vi "Begin.vi"() -> (0 "error out":errorcluster)   [LabVIEW 2013]
doc: "Called before other user functions, this VI is expected to open initial I/O refnums, load in file data, and do all program initialization. Notice that the <B>error out</B> terminal is simply used for data flow. Wiring it to other structures or subVIs ensures that this VI runs first."
uses:
  <vilib>/Rock Robotics/WPI/DriverStation/WPI_DriverStationRobotMode2.ctl
  DBNameEnum.ctl
  <vilib>/Rock Robotics/WPI/SafetyOutput/WPI_SafetyOutputConfigMenu.ctl
  <vilib>/Rock Robotics/WPI/Joystick/WPI_JoystickDeviceEnum.ctl
  RefnameEnum.ctl
  SingleSolenoidAction.ctl
  RollerAction.ctl
  TankDriveAction.ctl
  DoubleSolenoidAction.ctl
  CollectorAction.ctl
  <vilib>/Rock Robotics/WPI/Solenoid/WPI_SolenoidChannel.ctl
  <vilib>/Rock Robotics/SystemInterfaces/Typedef/FPGA_TypedefSolenoidModule.ctl
  <vilib>/Rock Robotics/SystemInterfaces/DIO/FPGA_DIOPWMChannel.ctl
  <vilib>/Rock Robotics/SystemInterfaces/Typedef/FPGA_TypedefDigitalModule.ctl
  <vilib>/Rock Robotics/SystemInterfaces/DIO/FPGA_DIOChannel.ctl
  <vilib>/Rock Robotics/SystemInterfaces/DIO/FPGA_DIORelayChannel.ctl
  <vilib>/Rock Robotics/WPI/Relay/WPI_RelayDirection.ctl
  <vilib>/Rock Robotics/SystemInterfaces/AI/FPGA_AIChannel.ctl
  SonarAction.ctl
  <vilib>/Rock Robotics/SystemInterfaces/Typedef/FPGA_TypedefAnalogModule.ctl
  Example_Code/PressureSensor/PressureSensorAction.ctl
  Robot Global Data.vi
  <vilib>/Rock Robotics/WPI/Solenoid/WPI_SolenoidOpenSingle.vi
  <vilib>/Rock Robotics/WPI/MotorControl/WPI_MotorControlOpen Talon.vi
  <vilib>/Rock Robotics/WPI/RobotDrive/WPI_RobotDriveOpen4MotorWithTalon.vi
  <vilib>/Rock Robotics/WPI/Compressor/WPI_CompressorGetSetRefNum.vi
panel:
  in  "Version":string="TF 2.3.2"
  # "SET AS DEFAULT"
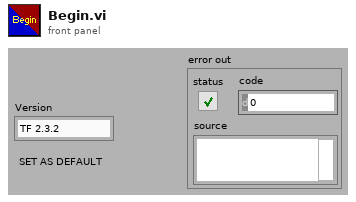
[diagram p1: front panel]
types:
  T1 = typedef "PressureSensorAction.ctl" = enum16{"Init", "ReadValue", "Disable"}
  T2 = typedef "FPGA_AIChannel.ctl" = enum8{"AI 1", "AI 2", "AI 3", "AI 4", "AI 5", "AI 6", "AI 7", "AI 8", "Invalid"}
  T3 = typedef "FPGA_TypedefAnalogModule.ctl" = enum16{"Analog Module 1", "Analog Module 2"}
  T4 = typedef "FPGA_DIOChannel.ctl" = enum8{"DIO 1", "DIO 2", "DIO 3", "DIO 4", "DIO 5", "DIO 6", "DIO 7", "DIO 8", "DIO 9", "DIO 10", "DIO 11", "DIO 12", "DIO 13", "DIO 14", "Invalid"}
  T5 = typedef "FPGA_DIOPWMChannel.ctl" = enum8{"PWM 1", "PWM 2", "PWM 3", "PWM 4", "PWM 5", "PWM 6", "PWM 7", "PWM 8", "PWM 9", "PWM 10", "Invalid"}
  T6 = typedef "SonarAction.ctl" = enum16{"Init", "ReadValue", "Disable"}
  T7 = typedef "WPI_RelayDirection.ctl" = enum16{"Both directions", "Forward only", "Reverse only"}
  T8 = typedef "FPGA_DIORelayChannel.ctl" = enum8{"Relay 1", "Relay 2", "Relay 3", "Relay 4", "Relay 5", "Relay 6", "Relay 7", "Relay 8", "Invalid"}
  T9 = typedef "WPI_SolenoidChannel.ctl" = enum8{"Solenoid 1", "Solenoid 2", "Solenoid 3", "Solenoid 4", "Solenoid 5", "Solenoid 6", "Solenoid 7", "Solenoid 8", "Invalid"}
  T10 = typedef "FPGA_TypedefSolenoidModule.ctl" = enum16{"Solenoid Module 1", "Solenoid Module 2"}
  T11 = typedef "FPGA_TypedefDigitalModule.ctl" = enum16{"Digital Module 1", "Digital Module 2"}
  T12 = typedef "SingleSolenoidAction.ctl" = enum16{"Init", "SetState", "Disable"}
  T13 = typedef "CollectorAction.ctl" = enum16{"Init", "Raise", "Lower", "Stop", "GetStatus"}
  T14 = typedef "DoubleSolenoidAction.ctl" = enum16{"Init", "Middle", "In", "Out"}
  T15 = typedef "TankDriveAction.ctl" = enum16{"Init", "LinearDrive", "SetValue", "Disable"}
  T16 = typedef "RefnameEnum.ctl" = enum16{"TankDrive", "Controller1", "Controller2", "SonicShifter", "Compressor"}
  T17 = typedef "RollerAction.ctl" = enum16{"Init", "Off", "Forward", "Reverse"}
  T18 = typedef "WPI_JoystickDeviceEnum.ctl" = enum16{"USB 1", "USB 2", "USB 3", "USB 4", "Kinect 1", "Kinect 2"}
  T19 = typedef "WPI_SafetyOutputConfigMenu.ctl" = enum16{"Enable", "Disable"}
  T20 = typedef "DBNameEnum.ctl" = enum16{"Version"}
  T21 = typedef "WPI_DriverStationRobotMode2.ctl" = enum16{"Autonomous Disabled", "Autonomous Enabled", "Teleop Disabled", "Teleop Enabled", "Timeout", "Finish", "Test Disabled", "Test Enabled"}
  T22 = typedef "WPI_JoystickDevRef.ctl" = cluster{"Device":T18}
  T23 = typedef "WPI_RobotDriveDevRef.ctl" = cluster{"DevStatus":errorcluster, "Motors[]":T24[], "Square Inputs":bool, "Max Output":dbl, "Isochronous":bool}
  T24 = typedef "WPI_MotorControlDeviceRef.ctl" = cluster{"DeviceStatus":errorcluster, "Type":enum16{"PWM", "CAN"}, "PWM":cluster{"Digital Module":T11, "PWM Channel":T5, "DeadBand":T25}, "CAN":cluster{"Device Number":u8, "Control Mode":T26, "Semaphore":T27, "Max Vout":dbl}, "Invert":bool, "TransformRef":T28, "InvTransformRef":T28}
  T25 = typedef "WPI_PWMDeadband.ctl" = cluster{"Name":string, "maxPositivePwm":i32, "minPositivePwm":i32, "centerPwm":i32, "maxNegativePwm":i32, "minNegativePwm":i32, "angularRange":u16}
  T26 = typedef "WPI_CANJaguar_ControlMode.ctl" = enum8{"Percent VBus", "Current", "Speed", "Position", "Voltage"}
  T27 = typedef "Semaphore RefNum" = refnum<k1>
  T28 = typedef "WPI_PWMTransform_ConPane.ctl" = refnum<vi>
  T29 = typedef "WPI_SolenoidDevRef.ctl" = cluster{"DevStatus":errorcluster, "Solenoid Module":T10, "Forward Solenoid Channel":T9, "Reverse Solenoid Channel":T9}
  T30 = typedef "WPI_AnalogChannelDevRef.ctl" = cluster{"DevStatus":errorcluster, "Analog Module":T3, "Analog Channel":T2}
  T31 = typedef "WPI_DigitalInputDevRef.ctl" = cluster{"DevStatus":errorcluster, "DIO Channel":T4, "Digital Module":T11}
  T32 = typedef "WPI_CompressorDevRef.ctl" = cluster{"DevStatus":errorcluster, "DigitalInputDevRef":T31, "RelayDevRef":T33}
  T33 = typedef "WPI_RelayDevRef.ctl" = cluster{"DevStatus":errorcluster, "Relay Channel":T8, "Digital Module":T11, "Relay Direction":T7}
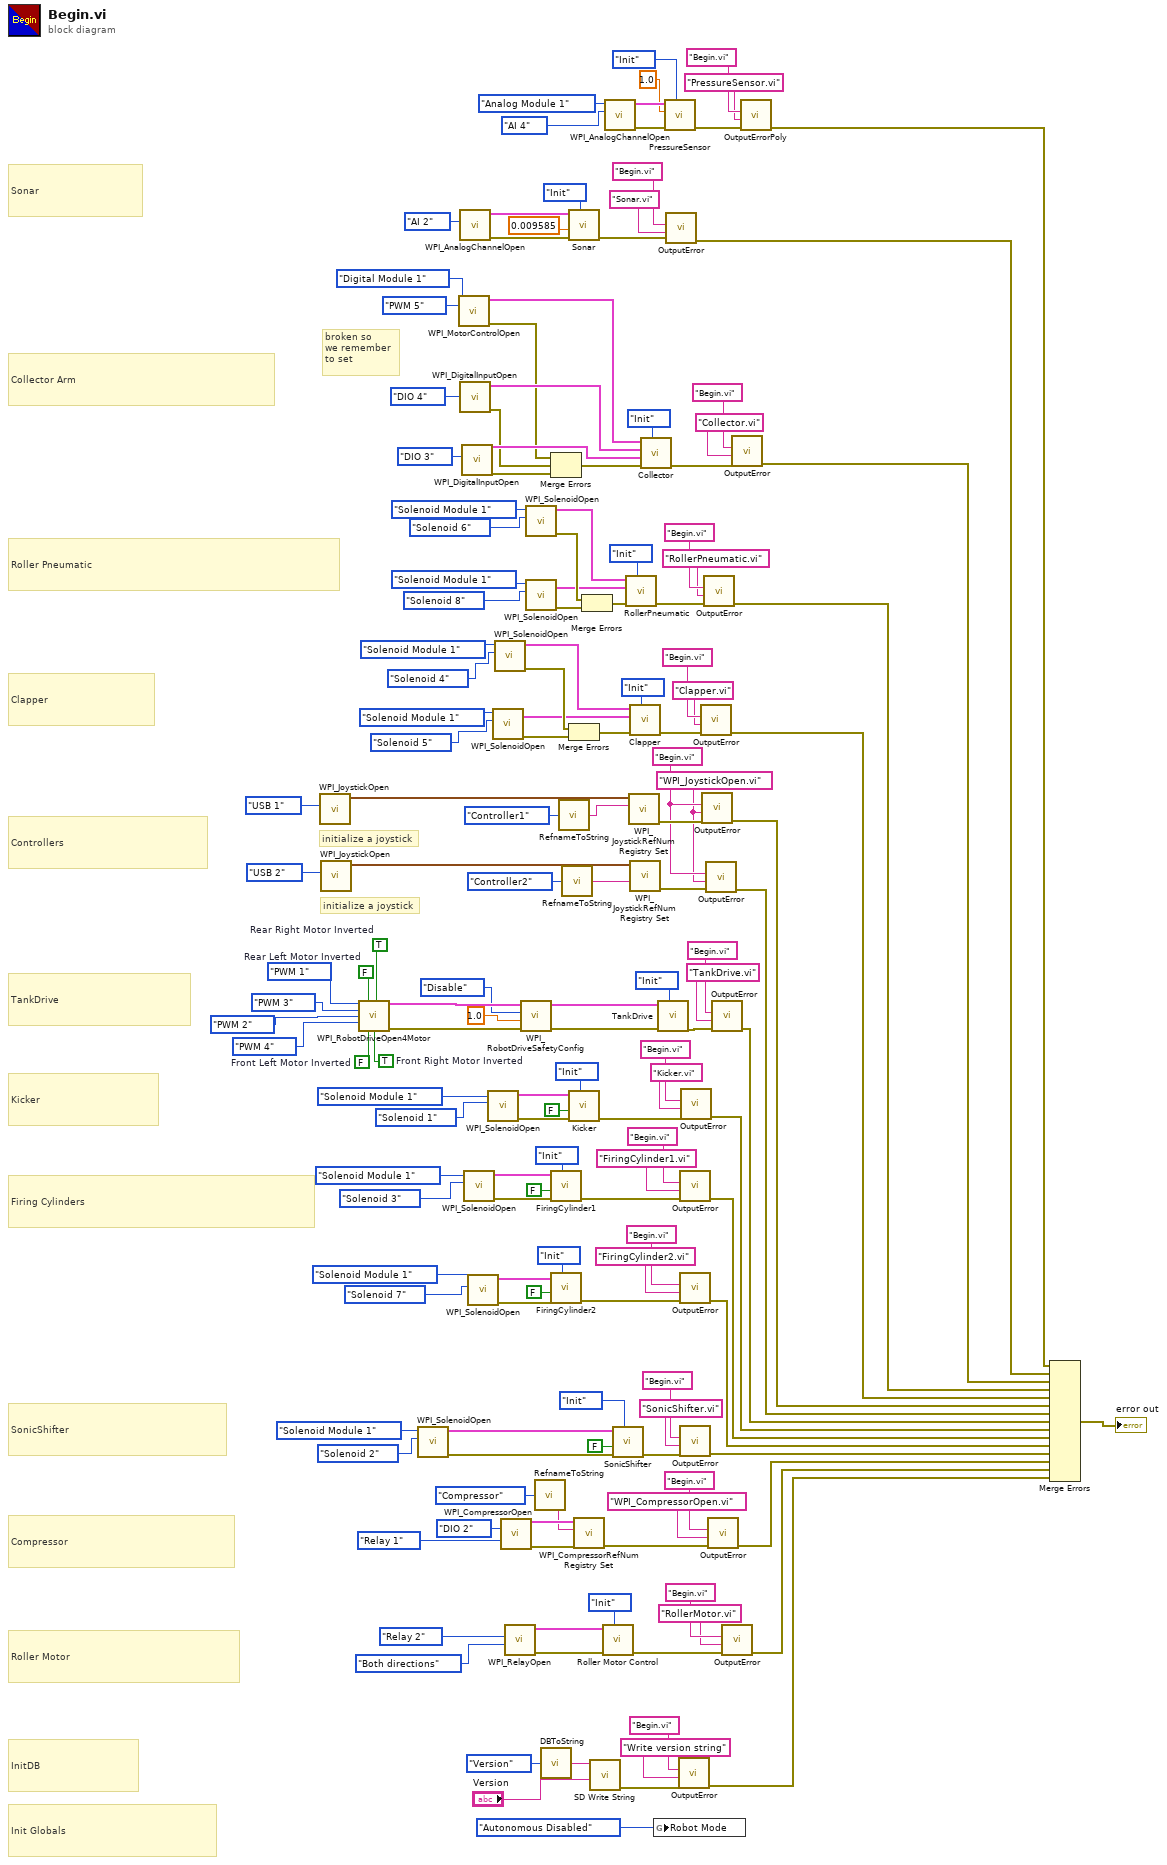
[diagram p0: block diagram]
diagram:
  w15 = TRUE  # Front Right Motor Inverted
  w16 = FALSE  # Front Left Motor Inverted
  w17 = TRUE  # Rear Right Motor Inverted
  w18 = FALSE  # Rear Left Motor Inverted
  w145 = "WPI_JoystickOpen.vi" ("Causing VI")
  w146 = "Begin.vi" ("Calling VI")
  # "broken so\nwe remember\nto set"
  # "Sonar"
  # "Collector Arm"
  # "Firing Cylinders"
  # "Roller Pneumatic"
  # "Clapper"
  # "Compressor"
  # "Roller Motor"
  # "SonicShifter"
  # "Controllers"
  # "initialize a joystick"
  # "initialize a joystick"
  # "TankDrive"
  # "Init Globals"
  # "InitDB"
  # "Kicker"
  n1 = call <vilib>:"WPI_JoystickOpen.vi"("JoystickDevice"=WPI_JoystickDeviceEnum."USB 1") -> ("JoystickDevRef"=w154:T22)  [unwired: 10 in]
  n2 = call <vilib>:"WPI_JoystickOpen.vi"("JoystickDevice"=WPI_JoystickDeviceEnum."USB 2") -> ("JoystickDevRef"=w151:T22)  [unwired: 10 in]
  n3 = call-poly <vilib>:"WPI_RobotDriveOpen4Motor.vi"("Rear Left Motor"=FPGA_DIOPWMChannel."PWM 1", "Rear Left Motor Inverted"=w18, "Rear Right Motor Inverted"=w17, "Rear Right Motor"=FPGA_DIOPWMChannel."PWM 3", "Front Left Motor"=FPGA_DIOPWMChannel."PWM 2", "Front Right Motor"=FPGA_DIOPWMChannel."PWM 4", "Front Left Motor Inverted"=w16, "Front Right Motor Inverted"=w15) -> ("RobotDriveDevRef"=w159:T23, "error out"=w158:errorcluster)  [unwired: 6 in]
  n4 = call-poly <vilib>:"WPI_SolenoidOpen.vi"("Solenoid Channel"=WPI_SolenoidChannel."Solenoid 2", "Solenoid Module (Module 1)"=FPGA_TypedefSolenoidModule."Solenoid Module 1") -> ("error out"=w101:errorcluster, "SolenoidDevRef"=w100:T29)  [unwired: 8 in]
  n5 = call-poly <vilib>:"WPI_MotorControlOpen.vi"("PWM Channel"=FPGA_DIOPWMChannel."PWM 5", "Digital Module (Module 1)"=FPGA_TypedefDigitalModule."Digital Module 1") -> ("error out"=w76:errorcluster, "MotorControlDeviceRef"=w82:T24)  [unwired: 8 in]
  n6 = call <vilib>:"WPI_AnalogChannelOpen.vi"("Analog Channel"=FPGA_AIChannel."AI 2") -> ("error out"=w30:errorcluster, "AIDeviceRef"=w31:T30)  [unwired: 9 in]
  n7 = call <vilib>:"WPI_DigitalInputOpen.vi"("DIO Channel"=FPGA_DIOChannel."DIO 4") -> ("error out"=w77:errorcluster, "DigitalInputDevRef"=w81:T31)  [unwired: 9 in]
  n8 = call <vilib>:"WPI_DigitalInputOpen.vi"("DIO Channel"=FPGA_DIOChannel."DIO 3") -> ("error out"=w78:errorcluster, "DigitalInputDevRef"=w80:T31)  [unwired: 9 in]
  n9 = call-poly <vilib>:"WPI_SolenoidOpen.vi"("Solenoid Channel"=WPI_SolenoidChannel."Solenoid 3", "Solenoid Module (Module 1)"=FPGA_TypedefSolenoidModule."Solenoid Module 1") -> ("error out"=w91:errorcluster, "SolenoidDevRef"=w90:T29)  [unwired: 8 in]
  n10 = call-poly <vilib>:"WPI_SolenoidOpen.vi"("Solenoid Channel"=WPI_SolenoidChannel."Solenoid 7", "Solenoid Module (Module 1)"=FPGA_TypedefSolenoidModule."Solenoid Module 1") -> ("error out"=w64:errorcluster, "SolenoidDevRef"=w63:T29)  [unwired: 8 in]
  n11 = call-poly <vilib>:"WPI_SolenoidOpen.vi"("Solenoid Channel"=WPI_SolenoidChannel."Solenoid 1", "Solenoid Module (Module 1)"=FPGA_TypedefSolenoidModule."Solenoid Module 1") -> ("error out"=w99:errorcluster, "SolenoidDevRef"=w96:T29)  [unwired: 8 in]
  n12 = call-poly <vilib>:"WPI_SolenoidOpen.vi"("Solenoid Channel"=WPI_SolenoidChannel."Solenoid 5", "Solenoid Module (Module 1)"=FPGA_TypedefSolenoidModule."Solenoid Module 1") -> ("error out"=w56:errorcluster, "SolenoidDevRef"=w55:T29)  [unwired: 8 in]
  n13 = call-poly <vilib>:"WPI_SolenoidOpen.vi"("Solenoid Channel"=WPI_SolenoidChannel."Solenoid 4", "Solenoid Module (Module 1)"=FPGA_TypedefSolenoidModule."Solenoid Module 1") -> ("error out"=w112:errorcluster, "SolenoidDevRef"=w111:T29)  [unwired: 8 in]
  n14 = call <vilib>:"WPI_CompressorOpen.vi"("Pressure Switch DIO Channel"=FPGA_DIOChannel."DIO 2", "Relay Channel"=FPGA_DIORelayChannel."Relay 1") -> ("CompressorDevRef"=w122:T32, "error out"=w121:errorcluster)  [unwired: 3 in, 9 out]
  n15 = call <vilib>:"WPI_RelayOpen.vi"("Relay Direction"=WPI_RelayDirection."Both directions", "Relay Channel"=FPGA_DIORelayChannel."Relay 2") -> ("error out"=w129:errorcluster, "RelayDevRef"=w127:T33)  [unwired: 8 in]
  n16 = call <vilib>:"WPI_RobotDriveSafetyConfig.vi"("error in (no error)"=w158, "timeout (s)"=1.0, "mode"=WPI_SafetyOutputConfigMenu."Disable", "RobotDriveDevRef"=w159) -> ("error out"=w1:errorcluster, "RobotDriveDevRef"=w2:T23)  [unwired: 6 in]
  n17 = call-poly <vilib>:"WPI_SolenoidOpen.vi"("Solenoid Channel"=WPI_SolenoidChannel."Solenoid 6", "Solenoid Module (Module 1)"=FPGA_TypedefSolenoidModule."Solenoid Module 1") -> ("error out"=w102:errorcluster, "SolenoidDevRef"=w103:T29)  [unwired: 8 in]
  n18 = call-poly <vilib>:"WPI_SolenoidOpen.vi"("Solenoid Channel"=WPI_SolenoidChannel."Solenoid 8", "Solenoid Module (Module 1)"=FPGA_TypedefSolenoidModule."Solenoid Module 1") -> ("error out"=w51:errorcluster, "SolenoidDevRef"=w50:T29)  [unwired: 8 in]
  n19 = call "RefnameToString.vi"("Enum"=RefnameEnum."Compressor") -> ("Refname"=w118:string)
  n20 = call "DBToString.vi"("Enum"=DBNameEnum."Version") -> ("Refname"=w161:string)
  n21 = Merge Errors(w76, w77, w78) -> (w79:errorcluster)
  n22 = call "FiringCylinder1.vi"("Action"=SingleSolenoidAction."Init", "error in (no error)"=w91, "Default Position"=FALSE, "SolenoidDevRef"=w90) -> ("error out"=w92:errorcluster)  [unwired: 7 in]
  n23 = call "FiringCylinder2.vi"("Action"=SingleSolenoidAction."Init", "error in (no error)"=w64, "Default Position"=FALSE, "SolenoidDevRef"=w63) -> ("error out"=w59:errorcluster)  [unwired: 7 in]
  n24 = call "RefnameToString.vi"("Enum"=RefnameEnum."Controller1") -> ("Refname"=w143:string)
  n25 = call "RefnameToString.vi"("Enum"=RefnameEnum."Controller2") -> ("Refname"=w141:string)
  n26 = call "Sonar.vi"("Action"=SonarAction."Init", "error in (no error)"=w30, "Scaling factor (V/in)"=0.009585, "AIDeviceRef"=w31) -> ("error out"=w26:errorcluster)  [unwired: 6 in, 1 out]
  n27 = Merge Errors(w112, w56) -> (w57:errorcluster)
  n28 = call "Kicker.vi"("Action"=SingleSolenoidAction."Init", "error in (no error)"=w99, "Default Position"=FALSE, "SolenoidDevRef"=w96) -> ("error out"=w98:errorcluster)  [unwired: 7 in]
  n29 = call <vilib>:"WPI_CompressorRefNum Registry Set.vi"("error in (no error)"=w121, "refnum name"=w118, "CompressorDevRef"=w122) -> ("error out"=w120:errorcluster)  [unwired: 7 in, 1 out]
  n30 = Merge Errors(w102, w51) -> (w52:errorcluster)
  n31 = call <vilib>:"SD Write String.vi"("String"="Version", "Name"=w161) -> ("error out"=w138:errorcluster)  [unwired: 8 in, 1 out]
  n32 = call "Roller Motor Control.vi"("Action"=RollerAction."Init" ("RollerState"), "Error in"=w129, "RelayDevRef"=w127) -> ("Error out"=w128:errorcluster)  [unwired: 8 in]
  n33 = call <vilib>:"WPI_AnalogChannelOpen.vi"("Analog Channel"=FPGA_AIChannel."AI 4", "Analog Module (Module 1)"=FPGA_TypedefAnalogModule."Analog Module 1") -> ("error out"=w10:errorcluster, "AIDeviceRef"=w9:T30)  [unwired: 8 in]
  n34 = call "SonicShifter.vi"("Action"=SingleSolenoidAction."Init" ("Mode"), "error in (no error)"=w101, "Default Position"=FALSE, "SolenoidDevRef"=w100) -> ("error out"=w137:errorcluster)  [unwired: 7 in]
  n35 = call "RollerPneumatic.vi"("State"=DoubleSolenoidAction."Init", "Error in"=w52, "Plugged"=w50, "Open"=w103) -> ("Error out"=w106:errorcluster)  [unwired: 7 in]
  n36 = call <vilib>:"WPI_JoystickRefNum Registry Set.vi"("refnum name"=w143, "JoystickDevRef"=w154) -> ("error out"=w147:errorcluster)  [unwired: 8 in, 1 out]
  n37 = call "Clapper.vi"("State"=DoubleSolenoidAction."Init", "Error in"=w57, "Plugged"=w55, "Open"=w111) -> ("Error out"=w110:errorcluster)  [unwired: 7 in]
  n38 = call <vilib>:"WPI_JoystickRefNum Registry Set.vi"("refnum name"=w141, "JoystickDevRef"=w151) -> ("error out"=w148:errorcluster)  [unwired: 8 in, 1 out]
  n39 = call "Collector.vi"("Action"=CollectorAction."Init", "Error in"=w79, "BottomLS"=w80, "TopLS"=w81, "Motor"=w82) -> ("Error out"=w84:errorcluster)  [unwired: 4 in, 2 out]
  n40 = global write "Robot Global Data.vi" "Robot Mode"(WPI_DriverStationRobotMode2."Autonomous Disabled" ("Robot Mode")) -> ()
  n41 = call "TankDrive.vi"("DriveAction"=TankDriveAction."Init", "error in (no error)"=w1, "RobotDriveDevRef"=w2) -> ("error out"=w155:errorcluster)  [unwired: 7 in, 1 out]
  n42 = call "PressureSensor.vi"("Action"=PressureSensorAction."Init", "error in (no error)"=w10, "PressureScaler"=1.0, "AIDeviceRef"=w9) -> ("error out"=w6:errorcluster)  [unwired: 6 in, 1 out]
  n43 = call "OutputError.vi"("error in (no error)"=w26, "Causing VI"="Sonar.vi", "Calling VI"="Begin.vi") -> ("error out"=w23:errorcluster)  [unwired: 8 in]
  n44 = call "OutputError.vi"("error in (no error)"=w138, "Causing VI"="Write version string", "Calling VI"="Begin.vi") -> ("error out"=w124:errorcluster)  [unwired: 8 in]
  n45 = call "OutputError.vi"("error in (no error)"=w92, "Causing VI"="FiringCylinder1.vi" ("Calling VI"), "Calling VI"="Begin.vi") -> ("error out"=w66:errorcluster)  [unwired: 8 in]
  n46 = call "OutputError.vi"("error in (no error)"=w59, "Causing VI"="FiringCylinder2.vi" ("Calling VI"), "Calling VI"="Begin.vi") -> ("error out"=w58:errorcluster)  [unwired: 8 in]
  n47 = call "OutputError.vi"("error in (no error)"=w137, "Causing VI"="SonicShifter.vi", "Calling VI"="Begin.vi") -> ("error out"=w136:errorcluster)  [unwired: 8 in]
  n48 = call "OutputError.vi"("error in (no error)"=w98, "Causing VI"="Kicker.vi" ("Calling VI"), "Calling VI"="Begin.vi") -> ("error out"=w67:errorcluster)  [unwired: 8 in]
  n49 = call "OutputError.vi"("error in (no error)"=w110, "Causing VI"="Clapper.vi", "Calling VI"="Begin.vi") -> ("error out"=w71:errorcluster)  [unwired: 8 in]
  n50 = call "OutputError.vi"("error in (no error)"=w147, "Causing VI"=w145, "Calling VI"=w146) -> ("error out"=w70:errorcluster)  [unwired: 8 in]
  n51 = call "OutputError.vi"("error in (no error)"=w106, "Causing VI"="RollerPneumatic.vi", "Calling VI"="Begin.vi") -> ("error out"=w72:errorcluster)  [unwired: 8 in]
  n52 = call "OutputError.vi"("error in (no error)"=w148, "Causing VI"=w145, "Calling VI"=w146) -> ("error out"=w69:errorcluster)  [unwired: 8 in]
  n53 = call "OutputError.vi"("error in (no error)"=w120, "Causing VI"="WPI_CompressorOpen.vi", "Calling VI"="Begin.vi") -> ("error out"=w117:errorcluster)  [unwired: 8 in]
  n54 = call "OutputError.vi"("error in (no error)"=w155, "Causing VI"="TankDrive.vi", "Calling VI"="Begin.vi") -> ("error out"=w68:errorcluster)  [unwired: 8 in]
  n55 = call "OutputError.vi"("error in (no error)"=w128, "Causing VI"="RollerMotor.vi", "Calling VI"="Begin.vi") -> ("error out"=w123:errorcluster)  [unwired: 8 in]
  n56 = call "OutputError.vi"("error in (no error)"=w84, "Causing VI"="Collector.vi", "Calling VI"="Begin.vi") -> ("error out"=w73:errorcluster)  [unwired: 8 in]
  n57 = call-poly "OutputErrorPoly.vi"("error in (no error)"=w6, "Causing VI"="PressureSensor.vi", "Calling VI"="Begin.vi") -> ("error out"=w5:errorcluster)  [unwired: 8 in]
  n58 = Merge Errors(w5, w23, w73, w72, w71, w70, w69, w68, w67, w66, w58, w136, w117, w123, w124) -> (→"error out":errorcluster)
